vi "Particle Analysis.vi"(8 "error in (no error)":errorcluster, 10 "LUT1":cluster{u16, u16}, 11 "Image in":T1) -> (0 "error out":errorcluster, 1 "Image Out":T1, 2 "Image Dst Out 2":T1, 3 "Image Dst Out 1":T1, 5 "Particle Measurements (Pixels)":dbl[][](array[numeric]))   [LabVIEW 2017]
uses:
  <vilib>/vision/Image Controls.llb/IMAQ Image.ctl
  <vilib>/vision/NI_Vision_Development_Module.lvlib
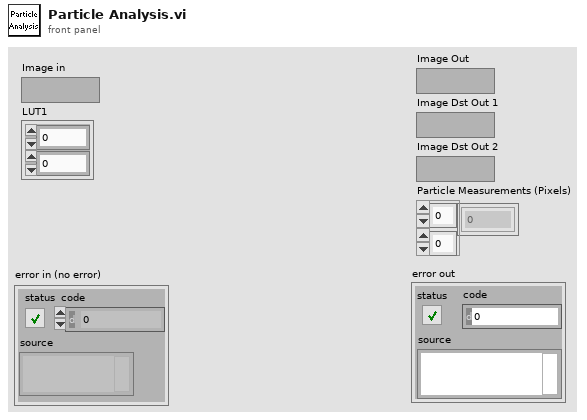
[diagram p1: front panel]
types:
  T1 = typedef "IMAQ Image.ctl" = refnum<image>
  T2 = enum32{"AutoM", "Close", "Dilate", "Erode", "Gradient", "Gradient out", "Gradient in", "Hit miss", "Open", "PClose", "POpen", "Thick", "Thin"}
  T3 = typedef "Particle Parameters" = i32
  T4 = typedef "Image Type" = u32
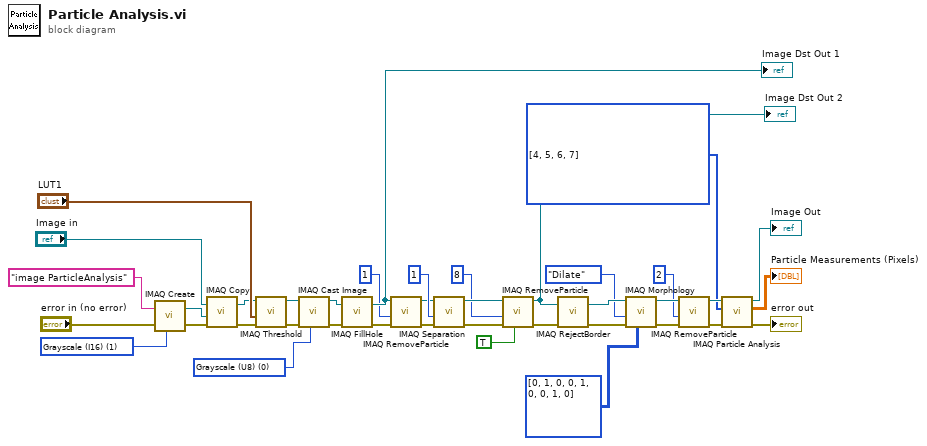
[diagram p0: block diagram]
diagram:
  w9 = T3[] [4, 5, 6, 7] items=["Center of Mass X", "Center of Mass Y", "First Pixel X", "First Pixel Y", "Bounding Rect Left", "Bounding Rect Top", "Bounding Rect Right", "Bounding Rect Bottom", "Max Feret Diameter Start X", "Max Feret Diameter Start Y", "Max Feret Diameter End X", "Max Feret Diameter End Y", "Max Horiz. Segment Length Left", "Max Horiz. Segment Length Right", "Max Horiz. Segment Length Row", "-", "Bounding Rect Width", "Bounding Rect Height", "Bounding Rect Diagonal", "Perimeter", "Convex Hull Perimeter", "Holes' Perimeter", "Max Feret Diameter", "Equivalent Ellipse Major Axis", "Equivalent Ellipse Minor Axis", "Equivalent Ellipse Minor Axis (Feret)", "Equivalent Rect Long Side", "Equivalent Rect Short Side", "Equivalent Rect Diagonal", "Equivalent Rect Short Side (Feret)", "Average Horiz. Segment Length", "Average Vert. Segment Length", "Hydraulic Radius", "Waddel Disk Diameter", "-", "Area", "Holes' Area", "Particle & Holes' Area", "Convex Hull Area", "Image Area", "-", "Number of Holes", "Number of Horiz. Segments", "Number of Vert. Segments", "-", "Orientation", "Max Feret Diameter Orientation", "-", "% Area/Image Area", "% Area/(Particle & Holes' Area)", "Ratio of Equivalent Ellipse Axes", "Ratio of Equivalent Rect Sides", "-", "Elongation Factor", "Compactness Factor", "Heywood Circularity Factor", "Type Factor", "-", "Sum X", "Sum Y", "Sum XX", "Sum XY", "Sum YY", "Sum XXX", "Sum XXY", "Sum XYY", "Sum YYY", "-", "Moment of Inertia XX", "Moment of Inertia XY", "Moment of Inertia YY", "Moment of Inertia XXX", "Moment of Inertia XXY", "Moment of Inertia XYY", "Moment of Inertia YYY", "Norm. Moment of Inertia XX", "Norm. Moment of Inertia XY", "Norm. Moment of Inertia YY", "Norm. Moment of Inertia XXX", "Norm. Moment of Inertia XXY", "Norm. Moment of Inertia XYY", "Norm. Moment of Inertia YYY", "Hu Moment 1", "Hu Moment 2", "Hu Moment 3", "Hu Moment 4", "Hu Moment 5", "Hu Moment 6", "Hu Moment 7"] ("Pixel Measurements")
  w7 = T4 0 items=["Grayscale (U8)", "Grayscale (I16)", "Grayscale (SGL)", "Complex (CSG)", "RGB (U32)", "HSL (U32)", "RGB (U64)", "Grayscale (U16)"] ("Image Type")
  w2 = T4 1 items=["Grayscale (U8)", "Grayscale (I16)", "Grayscale (SGL)", "Complex (CSG)", "RGB (U32)", "HSL (U32)", "RGB (U64)", "Grayscale (U16)"] ("Image Type")
  n1 = call "IMAQ Create"("Image Name"="image ParticleAnalysis", "Image Type"=w2, "error in (no error)"="error in (no error)") -> ("New Image"=w3:T1, "error out"=w28:errorcluster)  [unwired: 2 in]
  n2 = call "IMAQ Copy"("error in (no error)"=w28, "Image Dst"=w3, "Image Src"="Image in") -> ("error out"=w29:errorcluster, "Image Dst Out"=w5:T1)  [unwired: 3 in]
  n3 = call "IMAQ Threshold"("error in (no error)"=w29, "Range"="LUT1", "Image Src"=w5) -> ("error out"=w30:errorcluster, "Image Dst Out"=w24:T1)  [unwired: 3 in, 4 out]
  n4 = call "IMAQ Cast Image"("Image Type"=w7, "error in (no error)"=w30, "Image Src"=w24) -> ("error out"=w31:errorcluster, "Image Dst Out"=w25:T1)  [unwired: 7 in]
  n5 = call "IMAQ FillHole"("error in (no error)"=w31, "Image Src"=w25) -> ("error out"=w32:errorcluster, "Image Dst Out"=w26:T1)  [unwired: 4 in]
  "Image Dst Out 1" <- w26
  n6 = call "IMAQ RemoveParticle"("error in (no error)"=w32, "Number of Erosion"=1, "Image Src"=w26) -> ("error out"=w33:errorcluster, "Image Dst Out"=w11:T1)  [unwired: 4 in, 3 out]
  n7 = call "IMAQ Separation"("error in (no error)"=w33, "Nb of Erosion"=1, "Image Src"=w11) -> ("error out"=w34:errorcluster, "Image Dst Out"=w14:T1)  [unwired: 7 in]
  n8 = call "IMAQ RemoveParticle"("Low Pass/High Pass (Low)"=TRUE, "error in (no error)"=w34, "Number of Erosion"=8, "Image Src"=w14) -> ("error out"=w35:errorcluster, "Image Dst Out"=w16:T1)  [unwired: 3 in, 3 out]
  "Image Dst Out 2" <- w16
  n9 = call "IMAQ RejectBorder"("error in (no error)"=w35, "Image Src"=w16) -> ("error out"=w36:errorcluster, "Image Dst Out"=w18:T1)  [unwired: 4 in]
  n10 = call "IMAQ Morphology"("Structuring Element"=i32[][] [[0, 1, 0], [0, 1, 0], [0, 1, 0]], "error in (no error)"=w36, "Operation"=T2."Dilate", "Image Src"=w18) -> ("error out"=w37:errorcluster, "Image Dst Out"=w21:T1)  [unwired: 6 in]
  n11 = call "IMAQ RemoveParticle"("error in (no error)"=w37, "Number of Erosion"=2, "Image Src"=w21) -> ("error out"=w38:errorcluster, "Image Dst Out"=w22:T1)  [unwired: 4 in, 3 out]
  n12 = call "IMAQ Particle Analysis"("error in (no error)"=w38, "Pixel Measurements"=w9, "Image"=w22) -> ("error out"=→"error out":errorcluster, "Particle Measurements (Pixels)"=→"Particle Measurements (Pixels)":dbl[][], "Image Out (duplicate)"=→"Image Out":T1)  [unwired: 3 in, 3 out]
